vi "DSF.Engine.Framework.Get Runtime.vi"(8 "error in (no error)":errorcluster, 11 "Framework in":refnum<class "Framework.lvclass">) -> (0 "error out":errorcluster, 2 "Framework Runtime":refnum<class "DSF.Engine.Runtime.Framework.lvclass">, 3 "Framework out":refnum<class "Framework.lvclass">)   [LabVIEW 2016]
uses:
  Framework.lvclass
  DSF.Engine.Runtime.Framework.lvclass
  C:/Git/Sourcetree/DSF/Source/Engine/Classes/Runtime/DSF.Engine.Runtime.lvclass
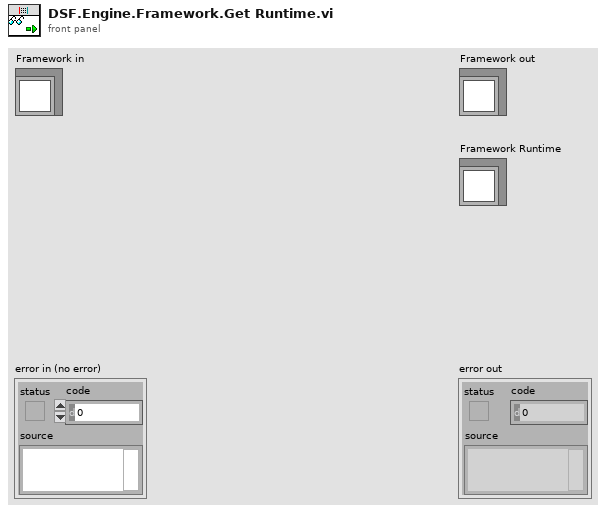
[diagram p1: front panel]
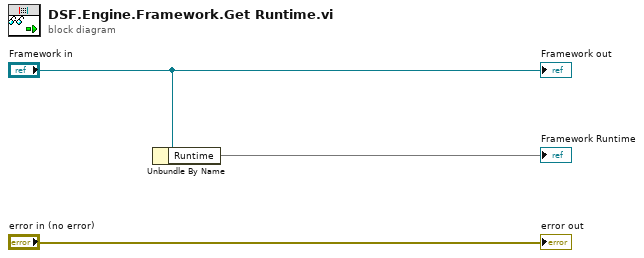
[diagram p0: block diagram]
diagram:
  n1 = Unbundle By Name("Framework in") -> ("Runtime"=→"Framework Runtime")
  "error out" <- "error in (no error)"
  "Framework out" <- "Framework in"
